vi "Get Telemetry Data.vi"(8 "error in (no error)":errorcluster, 10 "data":waveform(dbl)[](array[waveform]), 11 "TCP Network Connection in":refnum<k5>) -> (0 "error out":errorcluster, 2 "Telemetry Data":T1, 3 "TCP Network Connection out":refnum<k5>)   [LabVIEW 2026, in "TCP.lvlib"]
uses:
  Controls/Telemetry_Data_Type.ctl
  Controls/Channels.ctl
  Controls/Vibration_Data_Packet.ctl
  TCP.lvlib
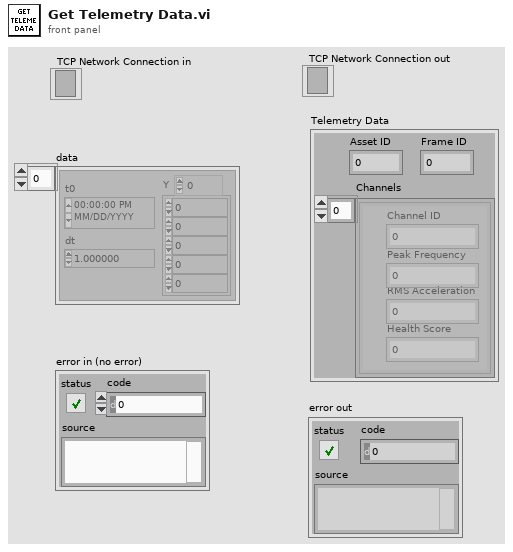
[diagram p1: front panel]
types:
  T1 = typedef "Telemetry_Data_Type.ctl" = cluster{"asset_id":i32, "channels":T2, "frame_id":i32}
  T2 = typedef "Channels.ctl" = cluster{"channel_id":dbl, "peak_frequency":dbl, "rms_acceleration":dbl, "health_score":dbl}[]
  T3 = typedef "Vibration_Data_Packet.ctl" = cluster{"sample_rate":dbl, "matrix":dbl[][]}
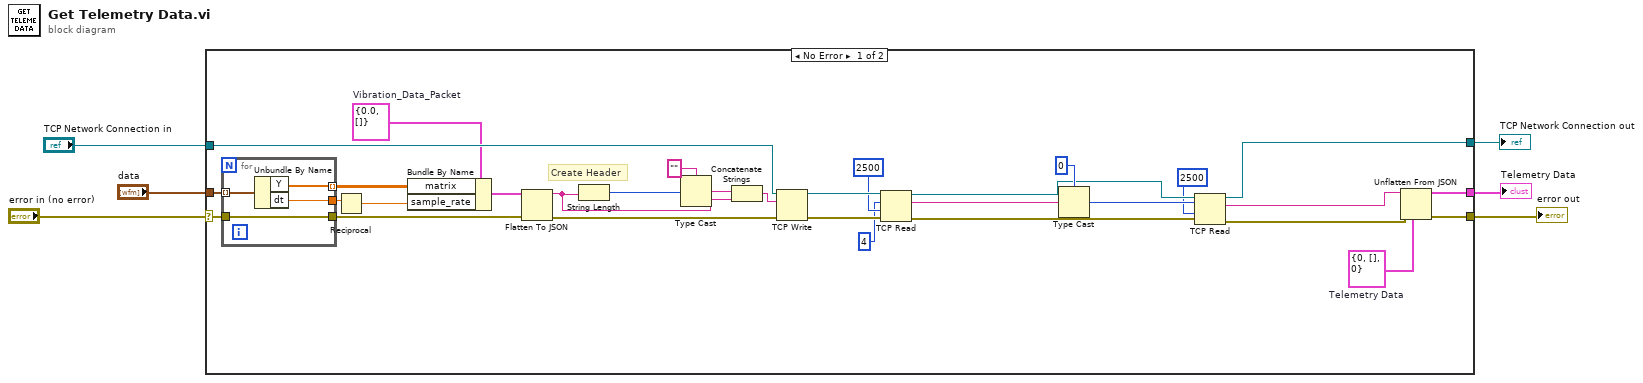
[diagram p0: block diagram]
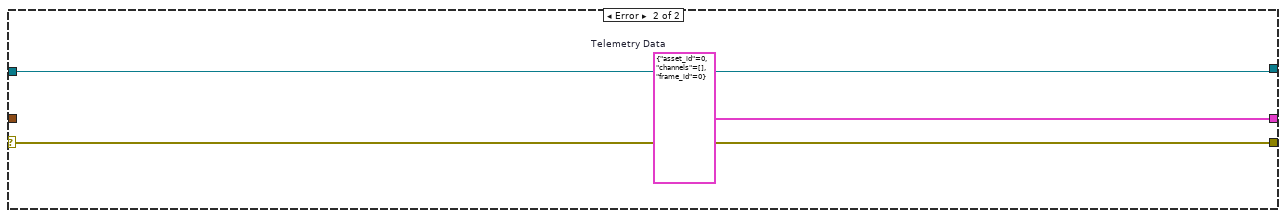
[diagram p2: hidden frame]
diagram:
  n1 = case shown="No Error" "error in (no error)" {
    selector: "error in (no error)" -> [w19 w44]
    tunnel: [w37 w43] -> w6
    tunnel: "TCP Network Connection in" -> [w30 w43]
    tunnel: "data" -> [w21 _]
    tunnel: [w20 w42] -> w1
    tunnel: [w18 w44] -> w2
    frame No Error {
      w14 = T3 {"sample_rate"=0.0, "matrix"=[]}  # Vibration_Data_Packet
      w17 = T1 {"asset_id"=0, "channels"=[], "frame_id"=0}  # Telemetry Data
      # "Create Header"
      n2 = for {
        tunnel: w19 -> [w39]
        tunnel: w21 -> [w41] mode=indexing
        tunnel: [w40] -> w12 mode=indexing
        tunnel: [w39] -> w22
        tunnel: [w38] -> w15
        n3 = Unbundle By Name(w41) -> ("Y"=w40:dbl[], "dt"=w38:dbl)
      }
      n4 = Reciprocal(x=w15) -> (1/x=w13:dbl)
      n5 = Bundle By Name(cluster=w14, "matrix"=w12, "sample_rate"=w13) -> (w11:T3)
      n6 = Flatten To JSON(anything=w11, error in (no error)=w22) -> (JSON string=w23:string, 11:w27:errorcluster)  [unwired: 1 in]
      n7 = String Length(string=w23) -> (length=w10:i32)
      n8 = Type Cast(type="", x=w10) -> (*(type *) &x=w25:string)
      n9 = Concatenate Strings(w25, w23) -> (w26:string)
      n10 = TCP Write(connection ID=w30, data in=w26, error in (no error)=w27) -> (connection ID out=w29:refnum<k5>, error out=w28:errorcluster)  [unwired: 1 in, 1 out]
      n11 = TCP Read(connection ID=w29, bytes to read=4, error in (no error)=w28, 9:2500 ("timeout ms (25000)")) -> (connection ID out=w16:refnum<k5>, data out=w31:string, error out=w34:errorcluster)  [unwired: 1 in]
      n12 = Type Cast(type=0, x=w31) -> (*(type *) &x=w33:i32)
      n13 = TCP Read(connection ID=w16, bytes to read=w33, error in (no error)=w34, 9:2500 ("timeout ms (25000)")) -> (connection ID out=w37:refnum<k5>, data out=w36:string, error out=w35:errorcluster)  [unwired: 1 in]
      n14 = Unflatten From JSON(JSON string=w36, type and defaults=w17, error in (no error)=w35) -> (value=w20:T1, error out=w18:errorcluster)  [unwired: 4 in]
    }
    frame Error {
      w42 = T1 {"asset_id"=0, "channels"=[], "frame_id"=0}  # Telemetry Data
    }
  }
  "TCP Network Connection out" <- w6
  "error out" <- w2
  "Telemetry Data" <- w1
